vi "forloopStructureExample2.vi"() -> ()   [LabVIEW 2014]
panel:
  out "Output Array\nIndicator":dbl[](array[numeric])
  in  "Input Array\nControl":dbl[](array[numeric])
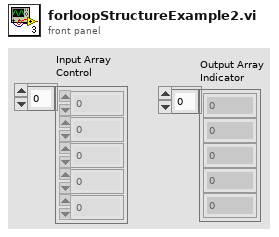
[diagram p1: front panel]
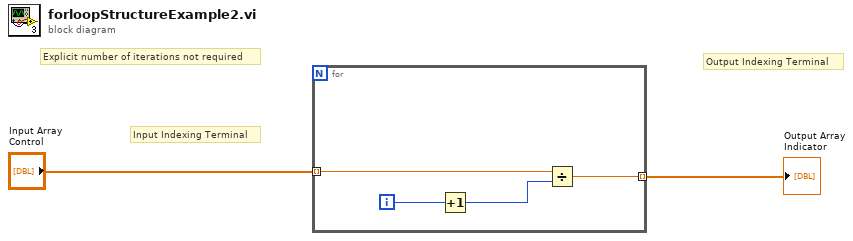
[diagram p0: block diagram]
diagram:
  # "Explicit number of iterations not required"
  # "Output Indexing Terminal"
  # "Input Indexing Terminal"
  n1 = for {
    tunnel: "Input Array\nControl" -> [w6] mode=indexing
    tunnel: [w5] -> w1 mode=indexing
    i -> [w4]
    n2 = Increment(x=w4) -> (x+1=w3:i32)
    n3 = Divide(x=w6, y=w3) -> (x/y=w5:dbl)
  }
  "Output Array\nIndicator" <- w1
